vi "1.3.vi"() -> ()   [LabVIEW 2013]
panel:
  out "element":string
  out "max value":dbl
  in  "Nombres":string[](array[string])
  in  "Edades":dbl[](array[numeric])
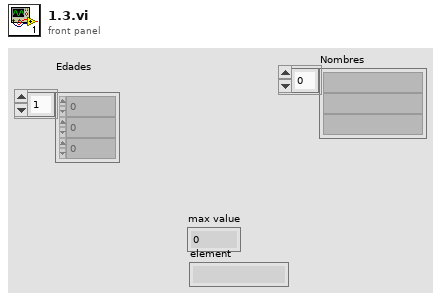
[diagram p1: front panel]
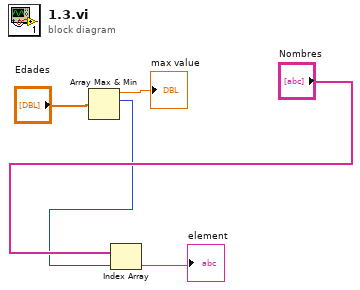
[diagram p0: block diagram]
diagram:
  n1 = Array Max & Min(array="Edades") -> (max value=→"max value":dbl, max index (indices)=w2:i32)  [unwired: 2 out]
  n2 = Index Array(array="Nombres", index=w2) -> (element=→"element":string)
